vi "InceptionTeleop2.vi"(6 "ZeroEncoder":bool=TRUE, 8 "Output":dbl format="%#_13g", 9 "MagicOutput":dbl format="%#_13g", 10 "StartMagic":bool, 11 "Talon #":string="Talon 2") -> ()   [LabVIEW 2017]
uses:
  <vilib>/Rock Robotics/WPI/ThirdParty/Phoenix-LabVIEW/Motor Controller/Controls/CTRE_Phoenix_MotorControl_FeedbackDevice.ctl
  <vilib>/Rock Robotics/WPI/ThirdParty/Phoenix-LabVIEW/Motor Controller/Controls/CTRE_Phoenix_MotorControl_ControlMode.ctl
panel:
  in  "F":dbl=0.0095 format="%#_13g"
  in  "D":dbl format="%#_13g"
  in  "I":dbl format="%#_13g"
  in  "P":dbl format="%#_13g"
  in  "Max Acceleration":i32=2000
  in  "Cruise Velocity":i32=2000
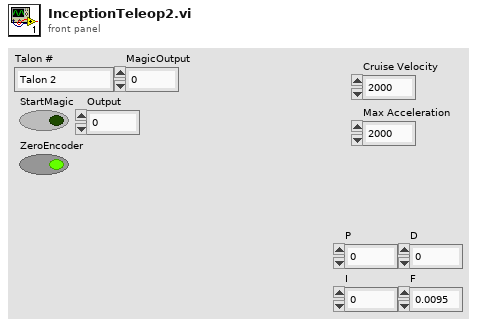
[diagram p1: front panel]
types:
  T1 = typedef "CTRE_Phoenix_MotorControl_FeedbackDevice.ctl" = i8
  T2 = typedef "WPI_MotorControlDeviceRef.ctl" = cluster{"DeviceStatus":errorcluster, "Type":T3, "PWM":cluster{"PWM Channel":T4, "DeadBand":T5}, "CAN":cluster{"Device Number":u8, "SetOutput VI Ref":variant, "GetOutput VI Ref":variant, "Enable VI Ref":variant, "Disable VI Ref":variant, "Data":variant}, "Invert":bool, "DIO PWM":cluster{"PWM \"Enable\" Channel":T4, "DIOChannel":T6, "PWM Rate":dbl}}
  T3 = typedef "WPI_MotorControlType.ctl" = enum16{"PWM", "CAN", "DIO PWM"}
  T4 = typedef "FPGA_DIOPWMChannel.ctl" = enum8{"PWM 0", "PWM 1", "PWM 2", "PWM 3", "PWM 4", "PWM 5", "PWM 6", "PWM 7", "PWM 8", "PWM 9", "PWM MXP 0", "PWM MXP 1", "PWM MXP 2", "PWM MXP 3", "PWM MXP 4", "PWM MXP 5", "PWM MXP 6", "PWM MXP 7", "PWM MXP 8", "PWM MXP 9", "Invalid"}
  T5 = typedef "WPI_PWMDeadband.ctl" = cluster{"Name":string, "maxPositivePwm":i32, "minPositivePwm":i32, "centerPwm":i32, "maxNegativePwm":i32, "minNegativePwm":i32, "angularRange":u16}
  T6 = typedef "FPGA_DIOChannel.ctl" = enum8{"DIO 0", "DIO 1", "DIO 2", "DIO 3", "DIO 4", "DIO 5", "DIO 6", "DIO 7", "DIO 8", "DIO 9", "DIO MXP 0", "DIO MXP 1", "DIO MXP 2", "DIO MXP 3", "DIO MXP 4", "DIO MXP 5", "DIO MXP 6", "DIO MXP 7", "DIO MXP 8", "DIO MXP 9", "DIO MXP 10", "DIO MXP 11", "DIO MXP 12", "DIO MXP 13", "DIO MXP 14", "DIO MXP 15", "SPI Port CS1", "SPI Port CS2", "SPI Port CS3", "SPI Port MISO", "SPI Port MOSI", "Invalid"}
  T7 = typedef "CTRE_Phoenix_MotorControl_ControlMode.ctl" = u16
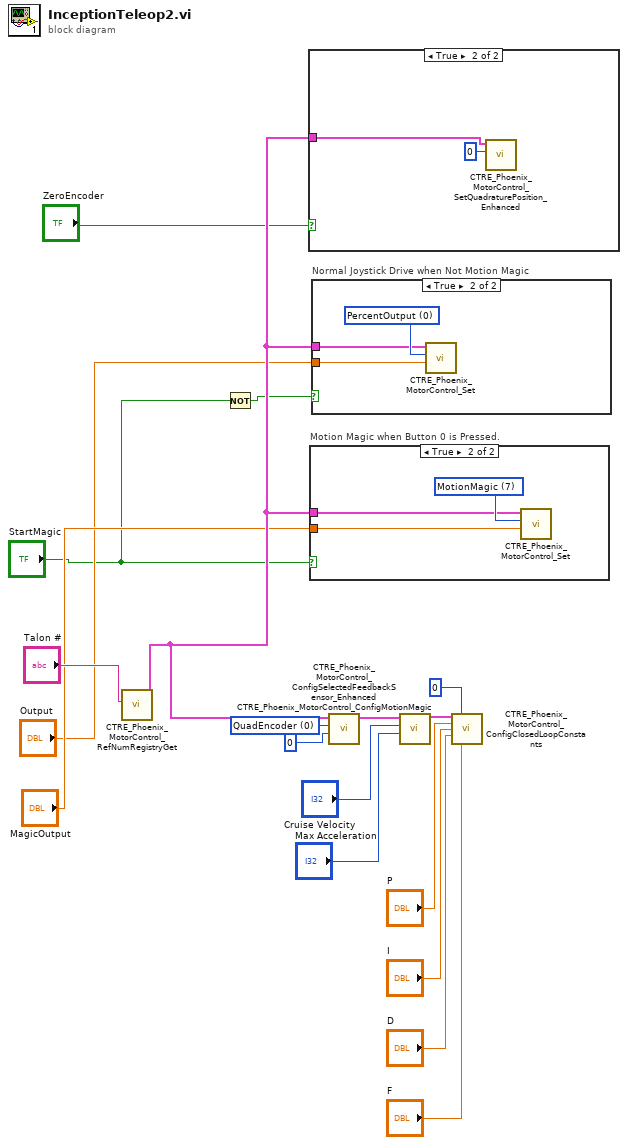
[diagram p0: block diagram]
diagram:
  w17 = T1 0 items=["None"=-1, "QuadEncoder"=0, "Analog"=2, "Tachometer"=4, "Pulse Width Encoded Position"=8, "Sensor Sum (S0 + S1)"=9, "Sensor Difference (D0 - D1)"=10, "Remote Source 0"=11, "Remote Source 1"=12, "Software Emulated"=15] ("Feedback Device")
  n1 = call <vilib>:"CTRE_Phoenix_MotorControl_RefNumRegistryGet.vi"("refnum name"="Talon #") -> ("PhoenixMotorControlDevRef"=w6:T2)  [unwired: 9 in, 1 out]
  n2 = Not(x="StartMagic") -> (.not. x?=w2:bool)
  n3 = case shown="True" "ZeroEncoder" {
    tunnel: w6 -> [_ w19]
    frame False {
    }
    frame True {
      n4 = call <vilib>:"CTRE_Phoenix_MotorControl_SetQuadraturePosition_Enhanced.vi"("New Position"=0, "PhoenixMotorControlDevRef"=w19) -> ()  [unwired: 8 in, 2 out]
    }
  }
  n5 = case "Motion Magic when Button 0 is Pressed." shown="True" "StartMagic" {
    tunnel: w6 -> [_ w22]
    tunnel: "MagicOutput" -> [_ w21]
    frame False {
    }
    frame True {
      w23 = T7 7 items=["PercentOutput"=0, "Position"=1, "Velocity"=2, "Follower"=5, "MotionProfile"=6, "MotionMagic"=7, "MotionMagicArc"=8, "TimedPercentOutput"=9, "Disabled"=15] ("Control Mode")
      n6 = call <vilib>:"CTRE_Phoenix_MotorControl_Set.vi"("Output"=w21, "Control Mode"=w23, "PhoenixMotorControlDevRef"=w22) -> ()  [unwired: 7 in, 2 out]
    }
  }
  n7 = case "Normal Joystick Drive when Not Motion Magic" shown="True" w2 {
    tunnel: w6 -> [_ w25]
    tunnel: "Output" -> [_ w24]
    frame False {
    }
    frame True {
      w26 = T7 0 items=["PercentOutput"=0, "Position"=1, "Velocity"=2, "Follower"=5, "MotionProfile"=6, "MotionMagic"=7, "MotionMagicArc"=8, "TimedPercentOutput"=9, "Disabled"=15] ("Control Mode")
      n8 = call <vilib>:"CTRE_Phoenix_MotorControl_Set.vi"("Output"=w24, "Control Mode"=w26, "PhoenixMotorControlDevRef"=w25) -> ()  [unwired: 7 in, 2 out]
    }
  }
  n9 = call <vilib>:"CTRE_Phoenix_MotorControl_ConfigSelectedFeedbackSensor_Enhanced.vi"("pidLoopIdx"=0, "Feedback Device"=w17, "PhoenixMotorControlDevRef"=w6) -> ("PhoenixMotorControlDevRef"=w16:T2)  [unwired: 7 in, 1 out]
  n10 = call <vilib>:"CTRE_Phoenix_MotorControl_ConfigMotionMagic.vi"("Acceleration"="Max Acceleration", "Cruise Velocity"="Cruise Velocity", "PhoenixMotorControlDevRef"=w16) -> ("PhoenixMotorControlDevRef"=w13:T2)  [unwired: 7 in, 1 out]
  n11 = call <vilib>:"CTRE_Phoenix_MotorControl_ConfigClosedLoopConstants.vi"("PhoenixMotorControlDevRef"=w13, "slotIdx"=0, "P"="P", "I"="I", "D"="D", "F"="F") -> ()  [unwired: 8 in, 2 out]
